vi "2D_interpolation.vi"(0 "X Axis Current":dbl[](array[numeric])=[-740.0, -570.0, -450.0, -340.0, -240.0, -150.0, -90.0, -30.0, 30.0, 90.0, 150.0, 240.0, 340.0, 450.0, 570.0, 740.0] format="%.2f", 1 "Min Z Value In":dbl format="%.2f", 5 "Y axis Current":dbl[](array[numeric])=[0.0, 1.0, 2.0, 3.0, 4.0] format="%.2f", 7 "Bkgnd Value":dbl, 9 "Plot In":dbl[][](graph)=[[0.00729, 0.1932, 1.451, 8.716, 18.11, 23.03, 24.73, 25.78, 25.44, 25.13, 24.23, 19.22, 10.83, 2.468, 0.2041, 0.06197], [0.04411, 0.08454, 1.327, 8.642, 17.93, 24.19, 25.23, 26.19, 26.05, 25.99, 24.99, 18.91, 9.149, 2.415, 0.2169, 0.07351], [0.05478, 0.1242, 1.515, 6.946, 14.88, 20.98, 22.81, 24.04, 24.28, 23.16, 20.91, 14.16, 6.61, 1.632, 0.1789, 0.1022], [0.04013, 0.1423, 1.178, 4.932, 9.291, 12.85, 15.3, 17.51, 17.21, 15.68, 12.8, 8.551, 4.232, 1.222, 0.1313, 0.08755], [0.04404, 0.1138, 0.7891, 2.319, 4.114, 6.265, 7.369, 8.39, 7.964, 7.127, 5.656, 3.956, 2.019, 0.6129, 0.1615, 0.08441]], 11 "Increment Value":dbl=1.0 format="%.2f", 12 "Transpose":bool=TRUE, 13 "Point Size":i32) -> (2 "min Z value":dbl format="%.2f", 3 "max Z value":dbl format="%.2f", 8 "Increment Value Out":dbl, 10 "Axis info":T1 {"Z Min" format="%.2f"; "Z Max" format="%.2f"; "Y Values" format="%.2f"; "X Values" format="%.2f"; "Y Scale"."delta X" format="%.2f"; "Y Scale"."Xo" format="%.2f"; "X Scale"."delta X" format="%.2f"; "X Scale"."Xo" format="%.2f"; "Y Max" format="%.2f"; "X Max" format="%.2f"}, 14 "Plot Out":dbl[][](graph)=[[0.00729, 0.18153463174730816, 0.17352738437348433, 1.6752433719500537, 8.231465735195274, 17.570357598383207, 23.099772817121426, 25.58386930448374, 25.31727725753219, 24.28926231541072, 18.717383219374323, 10.355253339797807, 2.7760273383248344, 0.3109897541921306, 0.08276881403435009, 0.06197], [0.04411, 0.1361526368018142, 0.04039202183336771, 1.5611636795339547, 8.176972694107874, 17.32000974741714, 24.257541358764026, 25.949153465972987, 26.01802540761648, 25.060373307424115, 18.284750328365213, 8.689831176707928, 2.642937641487066, 0.43219350072447926, -0.019957690739617468, 0.07351], [0.05478, 0.03446320268089581, 0.2086595806581808, 1.6919212249796047, 6.580368005180591, 14.333585185483123, 21.06810094963999, 23.709254571137723, 24.04768940379576, 21.01660820522005, 13.60443428327954, 6.2766496258038735, 1.7988963349022484, 0.2952877651784204, 0.05436788410934033, 0.1022], [0.04013, 0.06419557464541133, 0.2035068586120256, 1.3118741659450193, 4.7061387064566835, 9.009825946069038, 12.927700276268434, 17.003135081884164, 16.83885730812343, 12.902263313363814, 8.246161922417906, 4.035269404379355, 1.329605659745338, 0.24574055091433544, 0.012829784119986217, 0.08755], [0.04404, 0.022691144295571734, 0.19102098261858932, 0.8525411026079828, 2.2353542219792946, 3.966676465246214, 6.305347763088489, 8.17672908183636, 7.7348668140659, 5.703994479070454, 3.8329088824353237, 1.9256956625267279, 0.6611488869641811, 0.20508248283573002, 0.10119553469307395, 0.08441]], 15 "Raw Interpolation":dbl[][](array[numeric]) format="%.2f")   [LabVIEW 2020]
uses:
  <vilib>/Analysis/NI_AALPro.lvlib
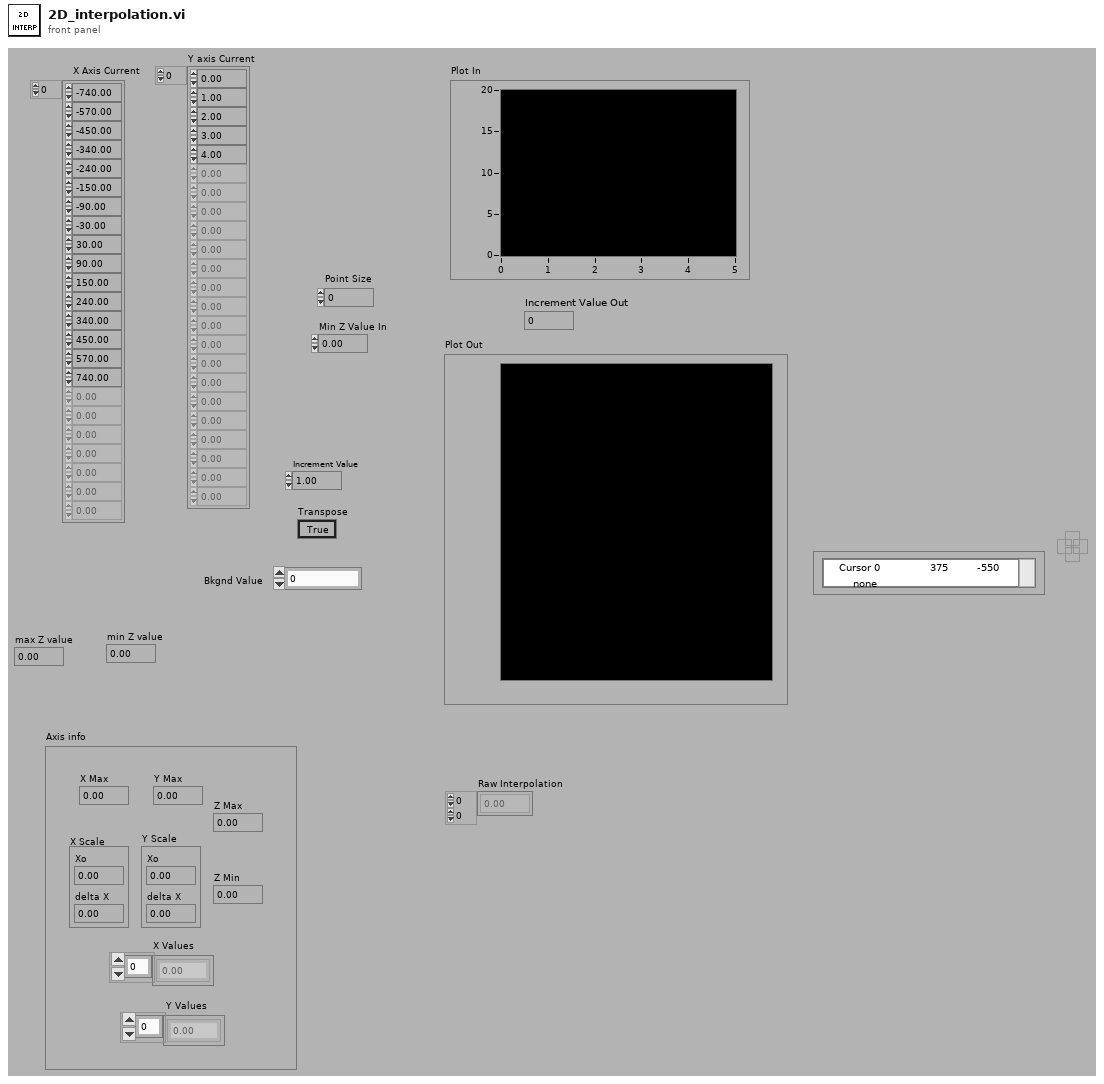
[diagram p1: front panel]
types:
  T1 = cluster{"X Max":dbl, "Y Max ":dbl, "X Scale":cluster{"Xo":dbl, "delta X":dbl}, "Y Scale":cluster{"Xo":dbl, "delta X":dbl}, "X Values":dbl[], "Y Values":dbl[], "Z Max":dbl, "Z Min":dbl}
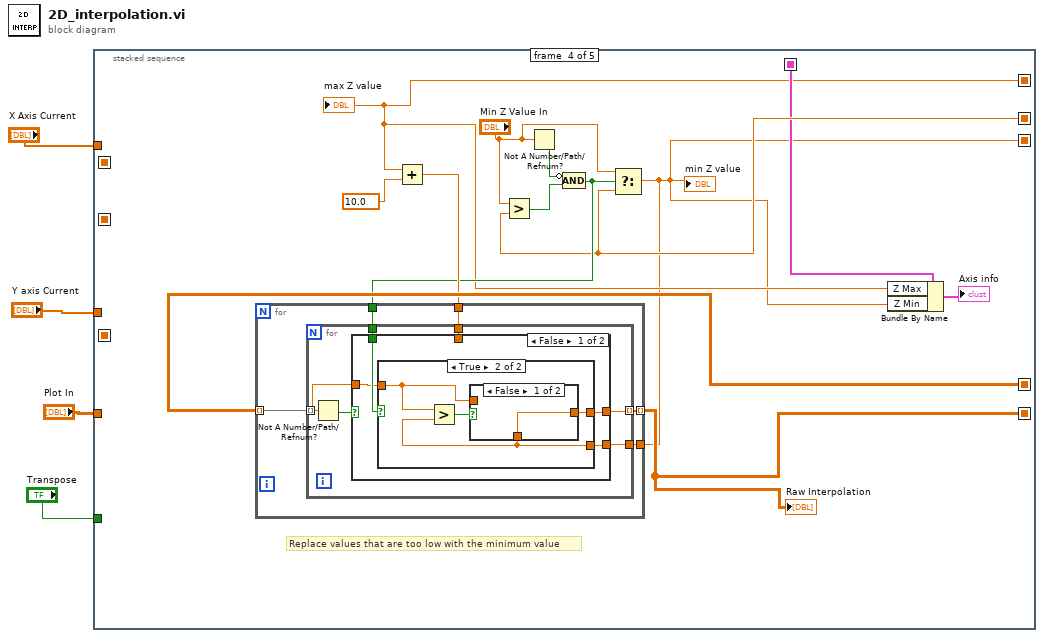
[diagram p0: block diagram]
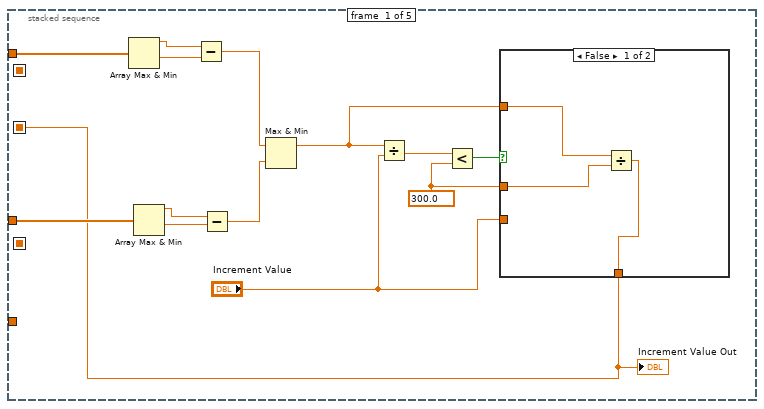
[diagram p2: hidden frame]
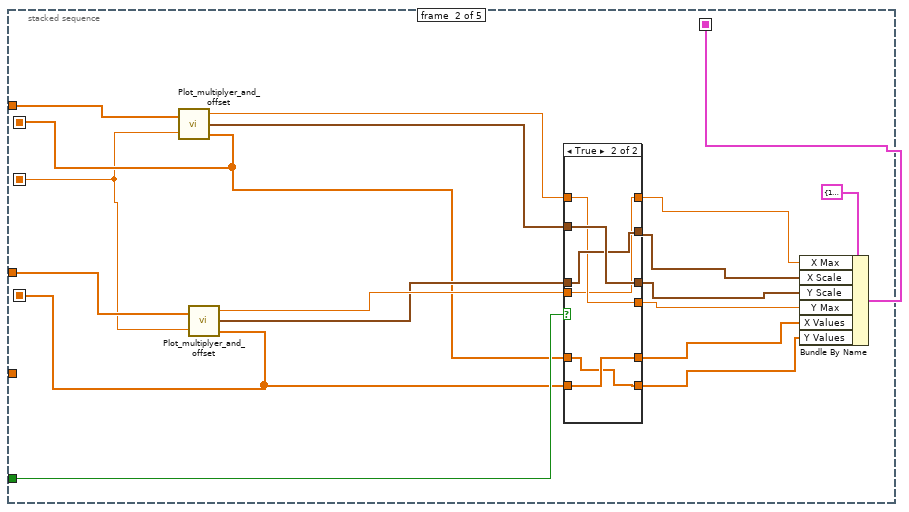
[diagram p4: hidden frame]
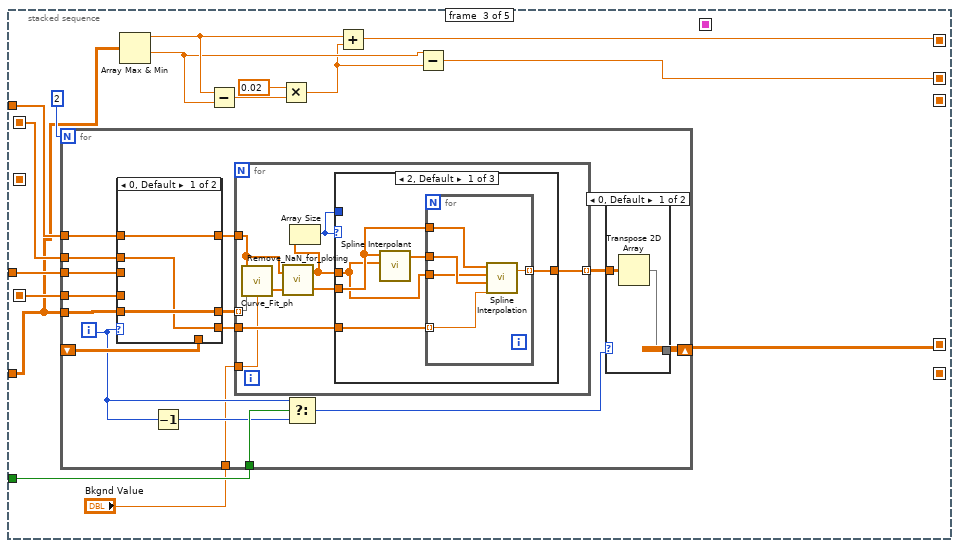
[diagram p6: hidden frame]
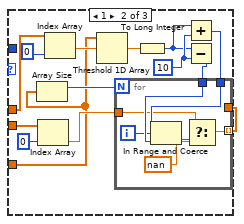
[diagram p9: hidden frame]
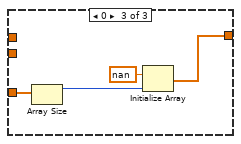
[diagram p10: hidden frame]
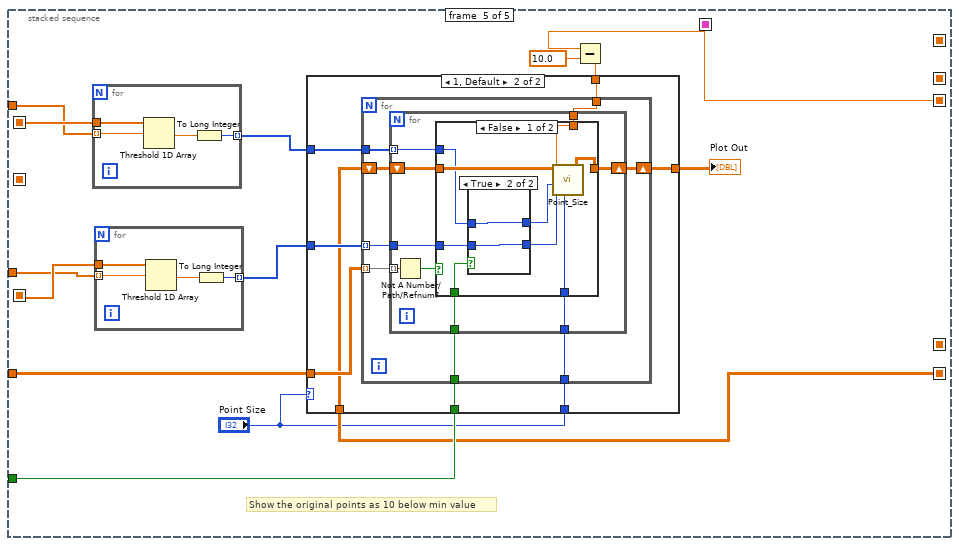
[diagram p14: hidden frame]
diagram:
  n1 = stacked-sequence {
    seq-local: [_ w33 _ _ _] -> [_ _ w66 _ w187]
    seq-local: [_ w32 _ _ _] -> [_ _ w64 _ w185]
    seq-local: [_ _ w62 _ _] -> [_ _ _ w150 _]
    seq-local: [_ _ w57 _ _] -> [_ _ _ w140 _]
    seq-local: [_ _ w54 _ _] -> [_ _ _ w143 _]
    seq-local: [_ _ _ w142 _] -> [_ _ _ _ w175]
    seq-local: [_ _ _ w139 _] -> [_ _ _ _ w176]
    seq-local: [w8 _ _ _ _] -> [_ w31 _ _ _]
    seq-local: [_ w23 _ _ _] -> [_ _ _ w141 _]
    tunnel: "X Axis Current" -> [w18 w39 w67 _ w186]
    tunnel: "Y axis Current" -> [w17 w36 w65 _ w184]
    tunnel: "Transpose" -> [_ w40 w63 _ w180]
    tunnel: "Plot In" -> [_ _ w61 _ w183]
    frame #0 {
      w5 = 300.0 ("y")
      n2 = Array Max & Min(array=w18) -> (max value=w16:dbl, min value=w15:dbl)  [unwired: 2 out]
      n3 = Array Max & Min(array=w17) -> (max value=w14:dbl, min value=w13:dbl)  [unwired: 2 out]
      n4 = Subtract(x=w16, y=w15) -> (x-y=w11:dbl)
      n5 = Subtract(x=w14, y=w13) -> (x-y=w12:dbl)
      n6 = Max & Min(x=w11, y=w12) -> (max(x,y)=w6:dbl)  [unwired: 1 out]
      n7 = Divide(x=w6, y="Increment Value") -> (x/y=w10:dbl)
      n8 = Less?(x=w10, y=w5) -> (x < y?=w9:bool)
      n9 = case shown="False" w9 {
        tunnel: [w19 w22] -> w8
        tunnel: "Increment Value" -> [_ w22]
        tunnel: w6 -> [w21 _]
        tunnel: w5 -> [w20 _]
        frame False {
          n10 = Divide(x=w21, y=w20) -> (x/y=w19:dbl)
        }
        frame True {
        }
      }
      "Increment Value Out" <- w8
    }
    frame #1 {
      n11 = call "Plot_multiplyer_and_offset.vi"("Position in"=w39, "Increment Value"=w31) -> ("Max Value"=w37:dbl, "Scale"=w38:cluster{"Xo":dbl, "delta X":dbl}, "Position Out"=w33:dbl[])
      n12 = call "Plot_multiplyer_and_offset.vi"("Position in"=w36, "Increment Value"=w31) -> ("Max Value"=w35:dbl, "Scale"=w34:cluster{"Xo":dbl, "delta X":dbl}, "Position Out"=w32:dbl[])
      n13 = case shown="True" w40 {
        tunnel: [w46 w51] -> w29
        tunnel: w38 -> [w46 w52]
        tunnel: [w45 w52] -> w28
        tunnel: w34 -> [w45 w51]
        tunnel: [w44 w49] -> w30
        tunnel: w37 -> [w44 w50]
        tunnel: [w43 w50] -> w27
        tunnel: w35 -> [w43 w49]
        tunnel: w33 -> [w42 w47]
        tunnel: [w42 w48] -> w26
        tunnel: w32 -> [w41 w48]
        tunnel: [w41 w47] -> w25
        frame False {
        }
        frame True {
        }
      }
      n14 = Bundle By Name(cluster=T1 {"X Max"=1450.0, "Y Max "=1500.0, "X Scale"={"Xo"=50.0, "delta X"=9.929078014184396}, "Y Scale"={"Xo"=-1500.0, "delta X"=9.966777408637874}, "X Values"=[50.0, 60.0, 70.0, 80.0, 90.0, 100.0, 110.0, 120.0, 130.0, 140.0, 150.0, 160.0, 170.0, 180.0, 190.0, 200.0, 210.0, 220.0, 230.0, 240.0, 250.0, 260.0, 270.0, 280.0, 290.0, 300.0, 310.0, 320.0, 330.0, 340.0, 350.0, 360.0, 370.0, 380.0, 390.0, 400.0, 410.0, 420.0, 430.0, 440.0, 450.0, 460.0, 470.0, 480.0, 490.0, 500.0, 510.0, 520.0, 530.0, 540.0, 550.0, 560.0, 570.0, 580.0, 590.0, 600.0, 610.0, 620.0, 630.0, 640.0, 650.0, 660.0, 670.0, 680.0, 690.0, 700.0, 710.0, 720.0, 730.0, 740.0, 750.0, 760.0, 770.0, 780.0, 790.0, 800.0, 810.0, 820.0, 830.0, 840.0, 850.0, 860.0, 870.0, 880.0, 890.0, 900.0, 910.0, 920.0, 930.0, 940.0, 950.0, 960.0, 970.0, 980.0, 990.0, 1000.0, 1010.0, 1020.0, 1030.0, 1040.0, 1050.0, 1060.0, 1070.0, 1080.0, 1090.0, 1100.0, 1110.0, 1120.0, 1130.0, 1140.0, 1150.0, 1160.0, 1170.0, 1180.0, 1190.0, 1200.0, 1210.0, 1220.0, 1230.0, 1240.0, 1250.0, 1260.0, 1270.0, 1280.0, 1290.0, 1300.0, 1310.0, 1320.0, 1330.0, 1340.0, 1350.0, 1360.0, 1370.0, 1380.0, 1390.0, 1400.0, 1410.0, 1420.0, 1430.0, 1440.0, 1450.0], "Y Values"=[-1500.0, -1490.0, -1480.0, -1470.0, -1460.0, -1450.0, -1440.0, -1430.0, -1420.0, -1410.0, -1400.0, -1390.0, -1380.0, -1370.0, -1360.0, -1350.0, -1340.0, -1330.0, -1320.0, -1310.0, -1300.0, -1290.0, -1280.0, -1270.0, -1260.0, -1250.0, -1240.0, -1230.0, -1220.0, -1210.0, -1200.0, -1190.0, -1180.0, -1170.0, -1160.0, -1150.0, -1140.0, -1130.0, -1120.0, -1110.0, -1100.0, -1090.0, -1080.0, -1070.0, -1060.0, -1050.0, -1040.0, -1030.0, -1020.0, -1010.0, -1000.0, -990.0, -980.0, -970.0, -960.0, -950.0, -940.0, -930.0, -920.0, -910.0, -900.0, -890.0, -880.0, -870.0, -860.0, -850.0, -840.0, -830.0, -820.0, -810.0, -800.0, -790.0, -780.0, -770.0, -760.0, -750.0, -740.0, -730.0, -720.0, -710.0, -700.0, -690.0, -680.0, -670.0, -660.0, -650.0, -640.0, -630.0, -620.0, -610.0, -600.0, -590.0, -580.0, -570.0, -560.0, -550.0, -540.0, -530.0, -520.0, -510.0, -500.0, -490.0, -480.0, -470.0, -460.0, -450.0, -440.0, -430.0, -420.0, -410.0, -400.0, -390.0, -380.0, -370.0, -360.0, -350.0, -340.0, -330.0, -320.0, -310.0, -300.0, -290.0, -280.0, -270.0, -260.0, -250.0, -240.0, -230.0, -220.0, -210.0, -200.0, -190.0, -180.0, -170.0, -160.0, -150.0, -140.0, -130.0, -120.0, -110.0, -100.0, -90.0, -80.0, -70.0, -60.0, -50.0, -40.0, -30.0, -20.0, -10.0, 0.0, 10.0, 20.0, 30.0, 40.0, 50.0, 60.0, 70.0, 80.0, 90.0, 100.0, 110.0, 120.0, 130.0, 140.0, 150.0, 160.0, 170.0, 180.0, 190.0, 200.0, 210.0, 220.0, 230.0, 240.0, 250.0, 260.0, 270.0, 280.0, 290.0, 300.0, 310.0, 320.0, 330.0, 340.0, 350.0, 360.0, 370.0, 380.0, 390.0, 400.0, 410.0, 420.0, 430.0, 440.0, 450.0, 460.0, 470.0, 480.0, 490.0, 500.0, 510.0, 520.0, 530.0, 540.0, 550.0, 560.0, 570.0, 580.0, 590.0, 600.0, 610.0, 620.0, 630.0, 640.0, 650.0, 660.0, 670.0, 680.0, 690.0, 700.0, 710.0, 720.0, 730.0, 740.0, 750.0, 760.0, 770.0, 780.0, 790.0, 800.0, 810.0, 820.0, 830.0, 840.0, 850.0, 860.0, 870.0, 880.0, 890.0, 900.0, 910.0, 920.0, 930.0, 940.0, 950.0, 960.0, 970.0, 980.0, 990.0, 1000.0, 1010.0, 1020.0, 1030.0, 1040.0, 1050.0, 1060.0, 1070.0, 1080.0, 1090.0, 1100.0, 1110.0, 1120.0, 1130.0, 1140.0, 1150.0, 1160.0, 1170.0, 1180.0, 1190.0, 1200.0, 1210.0, 1220.0, 1230.0, 1240.0, 1250.0, 1260.0, 1270.0, 1280.0, 1290.0, 1300.0, 1310.0, 1320.0, 1330.0, 1340.0, 1350.0, 1360.0, 1370.0, 1380.0, 1390.0, 1400.0, 1410.0, 1420.0, 1430.0, 1440.0, 1450.0, 1460.0, 1470.0, 1480.0, 1490.0, 1500.0], "Z Max"=20.016929951832633, "Z Min"=19.34532003328487} ("Axis info"), "X Max"=w30, "X Scale"=w29, "Y Scale"=w28, "Y Max"=w27, "X Values"=w26, "Y Values"=w25) -> (w23:T1)
    }
    frame #2 {
      n15 = for {
        N: 2 -> [_]
        tunnel: w61 -> [w83]
        shift-right: [w80] -> w62
        shift-left: _ -> [w81]
        tunnel: w67 -> [w77]
        tunnel: w66 -> [w76]
        tunnel: w65 -> [w75]
        tunnel: w64 -> [w74]
        tunnel: w63 -> [w73]
        tunnel: "Bkgnd Value" -> [w69]
        i -> [w70]
        n16 = case shown="0, Default" w70 {
          tunnel: w83 -> [w90 _]
          tunnel: [w90 w93] -> w82
          tunnel: w81 -> [_ w93]
          tunnel: [w89 w92] -> w79
          tunnel: [w88 w91] -> w78
          tunnel: w77 -> [w89 _]
          tunnel: w76 -> [w88 _]
          tunnel: w75 -> [_ w92]
          tunnel: w74 -> [_ w91]
          frame 0, Default {
          }
          frame 1 {
          }
        }
        n17 = Decrement(x=w70) -> (x-1=w71:i32)
        n18 = for {
          tunnel: w82 -> [w97] mode=indexing
          tunnel: w79 -> [w95]
          tunnel: [w102] -> w84 mode=indexing
          tunnel: w78 -> [w101]
          tunnel: w69 -> [w94]
          n19 = call "Curve_Fit_ph.vi"("Bkgnd Value"=w94, "Values In"=w97, "Positions"=w95) -> ("Values Out"=w96:dbl[])  [unwired: 1 in, 1 out]
          n20 = call "Remove_NaN_for_ploting.vi"("Array 2"=w96, "Array 1"=w95) -> ("Array 2 Out"=w100:dbl[], "Array 1 Out"=w99:dbl[])
          n21 = Array Size(array=w99) -> (size(s)=w98:i32)
          n22 = case shown="2, Default" w98 {
            tunnel: [w106 w120 w137] -> w102
            tunnel: w101 -> [w105 w113 w135]
            tunnel: w100 -> [w104 w114 _]
            tunnel: w99 -> [w103 w124 _]
            tunnel: w98 -> [_ _ _]
            frame 2, Default {
              n23 = call <vilib>:"Spline Interpolant.vi"("X"=w103, "Y"=w104) -> ("Interpolant"=w107:dbl[])  [unwired: 2 in, 1 out]
              n24 = for {
                tunnel: w107 -> [w112]
                tunnel: w104 -> [w111]
                tunnel: w103 -> [w110]
                tunnel: [w109] -> w106 mode=indexing
                tunnel: w105 -> [w108] mode=indexing
                n25 = call <vilib>:"Spline Interpolation.vi"("x value"=w108, "Interpolant"=w112, "X"=w110, "Y"=w111) -> ("interpolation value"=w109:dbl)  [unwired: 1 out]
              }
            }
            frame 1 {
              w117 = 10 ("y")
              n26 = Array Size(array=w113) -> (size(s)=w115:i32)
              n27 = Index Array(array=w114, index=0 ("Index")) -> (element=w119:dbl)
              n28 = Index Array(array=w124, index=0 ("Index")) -> (element=w118:dbl)
              n29 = Threshold 1D Array(2:w118, 3:w113) -> (0:w123:dbl)  [unwired: 1 out]
              n30 = To Long Integer(number=w123) -> (32bit integer=w116:i32)
              n31 = Add(x=w116, y=w117) -> (x+y=w122:i32)
              n32 = Subtract(x=w116, y=w117) -> (x-y=w121:i32)
              n33 = for {
                N: w115 -> [_]
                tunnel: w122 -> [w133]
                tunnel: w121 -> [w132]
                tunnel: [w130] -> w120 mode=indexing
                tunnel: w119 -> [w129]
                i -> [w127]
                n34 = In Range and Coerce(upper limit=w133, x=w127, lower limit=w132) -> (In Range?=w131:bool)  [unwired: 1 out]
                n35 = Select(t=w129, s=w131, f=nan) -> (s? t:f=w130:dbl)
              }
            }
            frame 0 {
              n36 = Array Size(array=w135) -> (size(s)=w134:i32)
              n37 = Initialize Array(nan ("Element Data"), w134) -> (w137:dbl[])
            }
          }
        }
        n38 = Select(t=w70, s=w73, f=w71) -> (s? t:f=w72:i32)
        n39 = case shown="0, Default" w72 {
          tunnel: w84 -> [w86 w87]
          tunnel: [w85 w87] -> w80
          frame 0, Default {
            n40 = Transpose 2D Array(2D array=w86) -> (transposed array=w85:dbl[][])
          }
          frame 1 {
          }
        }
      }
      n41 = Array Max & Min(array=w61) -> (max value=w58:dbl, min value=w56:dbl)  [unwired: 2 out]
      n42 = Subtract(x=w58, y=w56) -> (x-y=w60:dbl)
      n43 = Multiply(x=0.02, y=w60) -> (x*y=w55:dbl)
      n44 = Add(x=w58, y=w55) -> (x+y=w57:dbl)
      n45 = Subtract(x=w56, y=w55) -> (x-y=w54:dbl)
    }
    frame #3 {
      # "Replace values that are too low with the minimum value"
      n46 = Add(x=w140, y=10.0) -> (x+y=w148:dbl)
      n47 = Greater?(x="Min Z Value In", y=w143) -> (0:w147:bool)
      n48 = Not A Number/Path/Refnum?(number/path/refnum="Min Z Value In") -> (NaN/Path/Refnum?=w146:bool)
      n49 = Compound Arithmetic op=AND(invert w146, w147) -> (w144:bool)
      n50 = Select(t="Min Z Value In", s=w144, f=w143) -> (s? t:f=w139:dbl)
      "min Z value" <- w139
      n51 = for {
        tunnel: w150 -> [w155] mode=indexing
        tunnel: w148 -> [w154]
        tunnel: [w153] -> w142 mode=indexing
        tunnel: w144 -> [w152]
        tunnel: w139 -> [w151]
        n52 = for {
          tunnel: w155 -> [w157] mode=indexing
          tunnel: w154 -> [w159]
          tunnel: [w160] -> w153 mode=indexing
          tunnel: w152 -> [w158]
          tunnel: w151 -> [w156]
          n53 = Not A Number/Path/Refnum?(number/path/refnum=w157) -> (NaN/Path/Refnum?=w161:bool)
          n54 = case shown="False" w161 {
            tunnel: [w162 w173] -> w160
            tunnel: w159 -> [_ w173]
            tunnel: w158 -> [w165 _]
            tunnel: w157 -> [w164 _]
            tunnel: w156 -> [w163 _]
            frame False {
              n55 = case shown="True" w165 {
                tunnel: w164 -> [w166 w168]
                tunnel: w163 -> [_ w167]
                tunnel: [w166 w169] -> w162
                frame False {
                }
                frame True {
                  n56 = Greater?(x=w168, y=w167) -> (0:w170:bool)
                  n57 = case shown="False" w170 {
                    tunnel: [w171 w172] -> w169
                    tunnel: w168 -> [_ w172]
                    tunnel: w167 -> [w171 _]
                    frame False {
                    }
                    frame True {
                    }
                  }
                }
              }
            }
            frame True {
            }
          }
        }
      }
      "Raw Interpolation" <- w142
      n58 = Bundle By Name(cluster=w141, "Z Max"=w140, "Z Min"=w139) -> (→"Axis info":T1)
      "max Z value" <- w140
    }
    frame #4 {
      # "Show the original points as 10 below min value"
      n59 = for {
        tunnel: w187 -> [w235]
        tunnel: w186 -> [w234] mode=indexing
        tunnel: [w232] -> w182 mode=indexing
        n60 = Threshold 1D Array(2:w234, 3:w235) -> (0:w233:dbl)  [unwired: 1 out]
        n61 = To Long Integer(number=w233) -> (32bit integer=w232:i32)
      }
      n62 = for {
        tunnel: w185 -> [w231]
        tunnel: w184 -> [w230] mode=indexing
        tunnel: [w228] -> w181 mode=indexing
        n63 = Threshold 1D Array(2:w230, 3:w231) -> (0:w229:dbl)  [unwired: 1 out]
        n64 = To Long Integer(number=w229) -> (32bit integer=w228:i32)
      }
      n65 = Subtract(x=w176, y=10.0) -> (x-y=w177:dbl)
      n66 = case shown="1, Default" "Point Size" {
        tunnel: w183 -> [_ w196]
        tunnel: w182 -> [_ w195]
        tunnel: w181 -> [_ w194]
        tunnel: w180 -> [_ w193]
        tunnel: [w188 w192] -> w179
        tunnel: w177 -> [_ w191]
        tunnel: w175 -> [w188 w190]
        tunnel: "Point Size" -> [_ w189]
        frame 0 {
        }
        frame 1, Default {
          n67 = for {
            tunnel: w196 -> [w204] mode=indexing
            shift-right: [w200] -> w192
            shift-left: w190 -> [w201]
            tunnel: w194 -> [w203] mode=indexing
            tunnel: w195 -> [w202]
            tunnel: w193 -> [w199]
            tunnel: w191 -> [w198]
            tunnel: w189 -> [w197]
            n68 = for {
              tunnel: w204 -> [w213] mode=indexing
              tunnel: w203 -> [w211]
              tunnel: w202 -> [w210] mode=indexing
              shift-right: [w209] -> w200
              shift-left: w201 -> [w208]
              tunnel: w199 -> [w207]
              tunnel: w198 -> [w206]
              tunnel: w197 -> [w205]
              n69 = Not A Number/Path/Refnum?(number/path/refnum=w213) -> (NaN/Path/Refnum?=w212:bool)
              n70 = case shown="False" w212 {
                tunnel: w211 -> [w217 _]
                tunnel: w210 -> [w216 _]
                tunnel: w208 -> [w222 w227]
                tunnel: [w221 w227] -> w209
                tunnel: w207 -> [w219 _]
                tunnel: w206 -> [w220 _]
                tunnel: w205 -> [w214 _]
                frame False {
                  n71 = case shown="True" w219 {
                    tunnel: [w224 w226] -> w218
                    tunnel: w217 -> [w223 w226]
                    tunnel: w216 -> [w224 w225]
                    tunnel: [w223 w225] -> w215
                    frame False {
                    }
                    frame True {
                    }
                  }
                  n72 = call "Point_Size.vi"("New Value"=w220, "Array In"=w222, "Index1"=w215, "Index2"=w218, "Size"=w214) -> ("Array Out"=w221:dbl[][])
                }
                frame True {
                }
              }
            }
          }
        }
      }
      "Plot Out" <- w179
    }
  }
